vi "运行实验.vi"   [LabVIEW 2018]
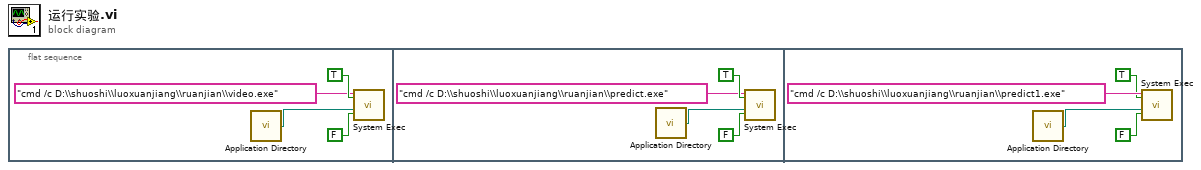
[diagram p0: block diagram]
diagram:
  n1 = flat-sequence {
    frame #0 {
      n2 = call <vilib>:"Application Directory.vi"() -> ("Application Directory"=w1:path)
      n3 = call <vilib>:"System Exec.vi"("run minimized? (F)"=FALSE, "wait until completion? (T)"=TRUE, "working directory"=w1, "command line"="cmd /c D:\\shuoshi\\luoxuanjiang\\ruanjian\\video.exe") -> ()  [unwired: 4 in, 4 out]
    }
    frame #1 {
      n4 = call <vilib>:"Application Directory.vi"() -> ("Application Directory"=w5:path)
      n5 = call <vilib>:"System Exec.vi"("run minimized? (F)"=FALSE, "wait until completion? (T)"=TRUE, "working directory"=w5, "command line"="cmd /c D:\\shuoshi\\luoxuanjiang\\ruanjian\\predict.exe" ("字符串")) -> ()  [unwired: 4 in, 4 out]
    }
    frame #2 {
      n6 = call <vilib>:"Application Directory.vi"() -> ("Application Directory"=w9:path)
      n7 = call <vilib>:"System Exec.vi"("run minimized? (F)"=FALSE, "wait until completion? (T)"=TRUE, "working directory"=w9, "command line"="cmd /c D:\\shuoshi\\luoxuanjiang\\ruanjian\\predict1.exe" ("字符串")) -> ()  [unwired: 4 in, 4 out]
    }
  }
